vi "Chamber controller Dec 14 2016.vi"() -> ()   [LabVIEW 2014]
uses:
  <vilib>/Instr/_visa.llb/VISA Configure Serial Port (Instr).vi
  Environmental Chamber LabVIEW and Instruments/Drivers and Software/Keithley 2100 Series/Public/Configure/Configure 2 Wire Resistance.vi
  <vilib>/Utility/file.llb/Write To Spreadsheet File (string).vi
  <vilib>/Utility/file.llb/Read From Spreadsheet File (string).vi
  Environmental Chamber LabVIEW and Instruments/Drivers and Software/keithley_6430/Keithley 6430/Public/Data/Read (Single Point).vi
  Environmental Chamber LabVIEW and Instruments/Drivers and Software/LabVIEW 8.2 Drivers/keithley_24xx/Keithley 24XX/Public/Data/Read (Single Point).vi
  Environmental Chamber LabVIEW and Instruments/Drivers and Software/keithley_24xx/Keithley 24XX/Keithley 24XX.lvlib
  Environmental Chamber LabVIEW and Instruments/Drivers and Software/keithley_6430/Keithley 6430/Keithley 6430.lvlib
  Environmental Chamber LabVIEW and Instruments/Drivers and Software/Keithley 2100 Series/Keithley 2100 Series.lvlib
panel:
  in  "Pressure parameters cluster":T1={"valve % open"=100.0, "Desired pressure"=0.0, "Vapor sccm"=0.0, "Gas sccm"=0.0, "Valve mode"=enum."% Open", "Pressure Mode"=enum."Abs. pressure", "analyte partial pressure"=23.8, "Turbo pump\nauto on"=TRUE, "Valve position (%)"=0.0, "read pressure"=0.0, "read vapor flow"=0.0, "read gas flow"=0.0} caption="Pressure settings" {"read gas flow" format="%#_3g"; "read vapor flow" format="%#_3g"; "read pressure" format="%#_7f"; "Valve position (%)" format="%#_3g"; "analyte partial pressure" min=0.0 max=100.0 step=5.0; "Gas sccm" min=0 max=200 step=5; "Vapor sccm" min=0 max=200 step=5; "Desired pressure" min=0.0 max=760.0 step=5.0; "valve % open" min=0.0 max=100.0 step=5.0 format="%#_2f"}
  out "pressure chart":cluster{"pressure":dbl}(graph)
  out "arduino qcm stack plot":T2(graph)
  in  "K-2420 tab control":enum32{"K-2420 Measure", "K-2420 Apply bias"}(tab)
  out "K-2420 2":cluster{"Resistance":sgl}(graph)
  in  "Bias (V)":dbl min=-5.0 max=5.0 step=5e-06
  out "K-2420 4":cluster{"Applied Voltage (V)":dbl}(graph)
  out "saving data?":bool
  in  "Data logging settings":T3={"Save during sequence only"=TRUE, "Save now"=FALSE, "sec between points"=0.0, "Current data file path"=path "", "Save sample/gas names"={"QCM1"="", "QCM2"="", "QCM3"="", "QCM4"="", "QCM5"="", "QCM6"="", "SRS"="bareAu", "K-2420"="", "K-6430"="", "K-2100"="", "Gas"="O2", "Vapor"="H2O"}, "add notes to file"=FALSE} {"sec between points" min=0.0 max=30.0 format="%#_13g"}
  in  "Sequence cluster":T4={"Save sequence"=FALSE, "Clear sequence"=FALSE, "Import sequence file"=FALSE, "Run Sequence"=FALSE, "Stop program when sequence ends"=TRUE, "User-defined\nsequence"=[], "Sequence end time"="", "Sequence\npreview"=[], "Current\nstep"=0, "Display"=0, "Sequence length (hrs)"=0.0} caption="Pressure settings" {"Display" items=["pressure", "gas flow", "vapor flow", "bias"]}
  out "J-KEM temp chart":dbl(graph)
  out "State date/time":string caption="Start time"
  out "K-2100 (Ohm)":cluster{"Measurement":dbl}(graph) caption="K-2100"
  out "K-6430":cluster{"Measurement":dbl}(graph)
  in  "Gate time (s)":enum16{"0.1", "1.0 ", "10"}(ring)=enum."1.0 "
  out "Hz":dbl format="%#.7f"
  out "QCM plot":T5(graph)
  in  "Stop":bool
  in  "Clear all charts":bool
  out "O2 sensor output":dbl[](array[numeric]) caption="atm\nTorr"
  in  "rapidox O2 Sensor":bool
  in  "setnag O2 Pump":bool
  in  "Baud Rate 2":i32(ring)=2 items=["2400", "4800", "9600", "19200", "38400", "57600", "115200"]
  in  "Com Port":i32(ring) items=["Com 1", "Com 2", "Com 3", "Com 4", "Com 5", "Com 6", "COM 7", "COM 8", "COM 9", "COM 10", "COM 11", "COM 12", "com 13", "COM 14"]
  in  "Com Port 2":i32(ring) items=["Com 1", "Com 2", "Com 3", "Com 4", "Com 5", "Com 6", "COM 7", "COM 8", "COM 9", "COM 10", "COM 11", "COM 12", "com 13", "COM 14"]
  out "Waveform Chart":cluster{dbl}(graph)
  out "O2 Concentration (PPM)":dbl
  out "Waveform Chart 6":cluster{dbl}(graph)
  # "SRS"
  # "Currently Unused"
  # "100%"
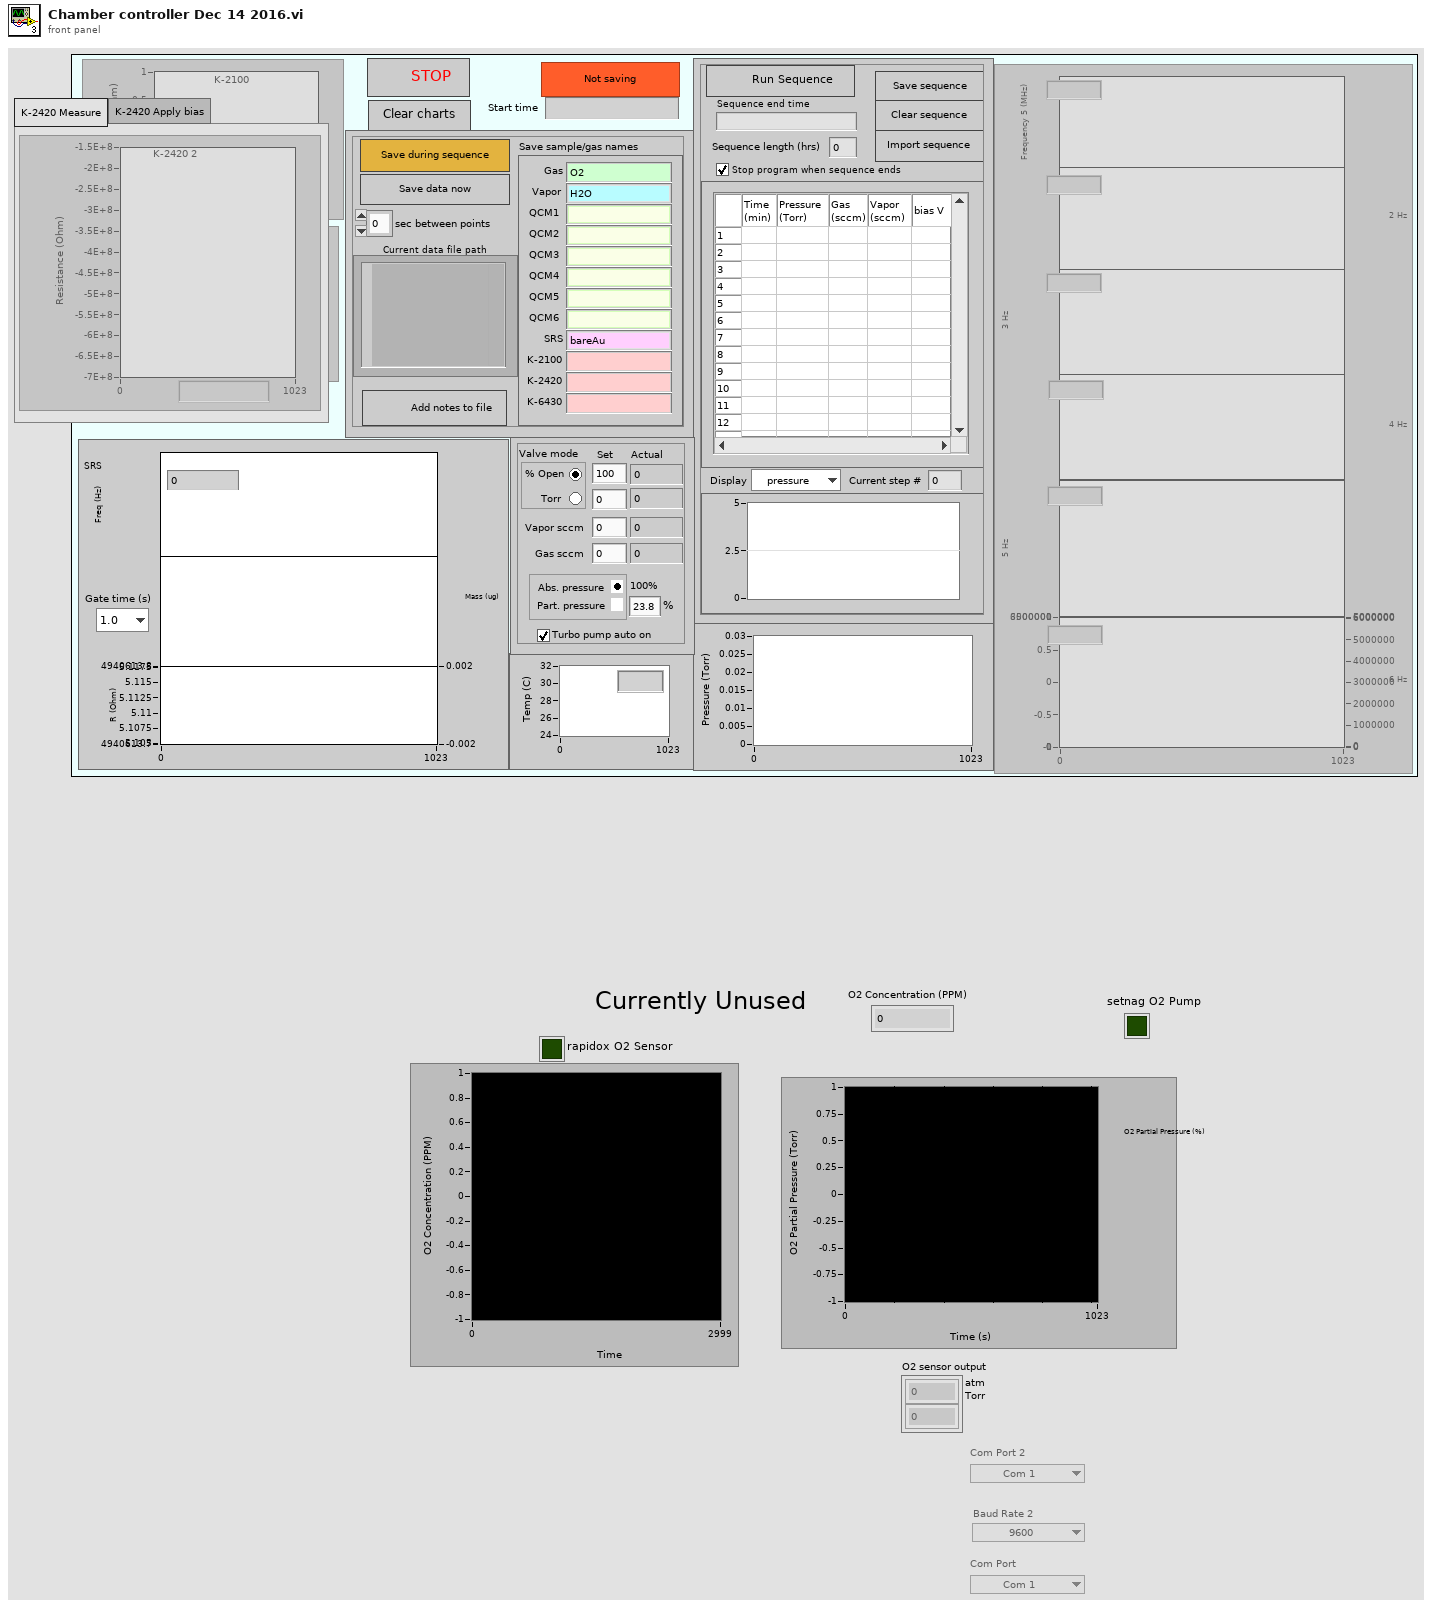
[diagram p1: front panel]
types:
  T1 = cluster{"valve % open":dbl, "Desired pressure":dbl, "Vapor sccm":sgl, "Gas sccm":sgl, "Valve mode":enum32{"% Open", "Torr "}, "Pressure Mode":enum32{"Abs. pressure", " Part. pressure"}, "analyte partial pressure":dbl, "Turbo pump\nauto on":bool, "Valve position (%)":dbl, "read pressure":dbl, "read vapor flow":dbl, "read gas flow":dbl}
  T2 = cluster{"mean":dbl, "mean":dbl, "mean":dbl, "mean":dbl, "mean":dbl, "mean":dbl}
  T3 = cluster{"Save during sequence only":bool, "Save now":bool, "sec between points":dbl, "Current data file path":path, "Save sample/gas names":cluster{"QCM1":string, "QCM2":string, "QCM3":string, "QCM4":string, "QCM5":string, "QCM6":string, "SRS":string, "K-2420":string, "K-6430":string, "K-2100":string, "Gas":string, "Vapor":string}, "add notes to file":bool}
  T4 = cluster{"Save sequence":bool, "Clear sequence":bool, "Import sequence file":bool, "Run Sequence":bool, "Stop program when sequence ends":bool, "User-defined\nsequence":string[][], "Sequence end time":string, "Sequence\npreview":cluster{dbl[], dbl[]}[], "Current\nstep":i32, "Display":u16, "Sequence length (hrs)":dbl}
  T5 = cluster{"Frequency out":dbl, "Numeric Control":dbl, "Resistance out":dbl}
  T6 = cluster{"Keithley 6430":bool, "J-KEM":bool, "Keithley 2420":bool, "Keithley 2100":bool, "SRS QCM":bool, "Pressure control":bool, "Arduino":bool}
  T7 = cluster{"Arduino 1":refnum<visa-resource-name>, "Arduino 2":refnum<visa-resource-name>, "Arduino 3":refnum<visa-resource-name>, "Arduino 4":refnum<visa-resource-name>, "Arduino 5":refnum<visa-resource-name>, "Arduino 6":refnum<visa-resource-name>}
  T8 = enum8{"Enabled", "Disabled", "Disabled and Grayed Out"}
  T9 = enum16{"open", "open or create", "create or replace", "create", "open (read only)"}
  T10 = enum16{"no parity", "odd parity", "even parity", "mark parity", "space parity"}
  T11 = cluster{"mean":dbl, "mean":dbl, "mean":dbl, "mean":dbl, "mean":dbl, "mean":dbl}[]
  T12 = cluster{"Frequency out":dbl, "Numeric Control":dbl, "Resistance out":dbl}[]
  T13 = cluster{"String":string, "String":string, "String":string}
  T14 = cluster{bool, "task out":refnum<k21>, "error out":errorcluster, "task out":refnum<k21>, "error out":errorcluster, "turbo pump":refnum<visa-resource-name>, "error out":errorcluster}
  T15 = cluster{bool, "task out":refnum<k21>, "error out":errorcluster, "task out":refnum<k21>, "error out":errorcluster, "VISA resource name out":refnum<visa-resource-name>, "error out":errorcluster}
  T16 = cluster{bool, "VISA resource name":refnum<visa-resource-name>, "error out":errorcluster}
  T17 = cluster{bool, "VISA resource name out":refnum<visa-resource-name>, "error out":errorcluster}
  T18 = cluster{"VISA resource name out":refnum<visa-resource-name>, "error out":errorcluster, "VISA resource name out":refnum<visa-resource-name>, "error out":errorcluster, "VISA resource name out":refnum<visa-resource-name>, "error out":errorcluster, "VISA resource name out":refnum<visa-resource-name>, "error out":errorcluster, "VISA resource name out":refnum<visa-resource-name>, "error out":errorcluster, "VISA resource name out 2":refnum<visa-resource-name>, "error out 2":errorcluster}
  T19 = cluster{"Boolean":bool, "VISA resource name out":refnum<visa-resource-name>, "error out":errorcluster}
  T20 = cluster{bool, "VISA out":refnum<visa-resource-name>, "error out":errorcluster}
  T21 = cluster{"Boolean":bool, "VISA out":refnum<visa-resource-name>, "error out":errorcluster}
  T22 = cluster{"Numeric Control":dbl, "Cluster":cluster{"Numeric Control":dbl}, "String":string, "error out":errorcluster}
  T23 = cluster{bool, "Com Port":i32, "Numeric Control out":dbl}
  T24 = cluster{"Arduino address":refnum<visa-resource-name>, "error in (no error)":errorcluster, "Arduino address 2":refnum<visa-resource-name>, "error in (no error) 2":errorcluster, "Arduino address 3":refnum<visa-resource-name>, "error in (no error) 3":errorcluster, "Arduino address 4":refnum<visa-resource-name>, "error in (no error) 4":errorcluster, "Arduino address 5":refnum<visa-resource-name>, "error in (no error) 5":errorcluster, "Arduino address 6":refnum<visa-resource-name>, "error in (no error) 6":errorcluster}
  T25 = cluster{"mean":string, "mean":string, "mean":string, "mean":string, "mean":string, "mean":string}
  T26 = cluster{"valve % open":dbl, "Desired pressure":dbl, "Vapor sccm":sgl, "Gas sccm":sgl, "Valve mode":enum32{"% Open", "Torr "}, "Pressure Mode":enum32{"Abs. pressure", " Part. pressure"}, "analyte partial pressure":dbl}
  T27 = cluster{"User-defined\nsequence":string[][], "Present (s)":dbl, "current  step # in":i32, "sequence end time in":timestamp}
  T28 = cluster{"current  step # in":i32, "sequence end time in":timestamp, "Boolean":bool}
  T29 = cluster{"press/RH/gas/vapor":cluster{"pressure":string, "RH":string, "gas flow":string, "vapor flow":string}, "Cluster":cluster{"Valve position (%)":dbl, "read pressure":dbl, "read vapor flow":dbl, "read gas flow":dbl}}
  T30 = cluster{"Boolean":bool, "task out":refnum<k21>, "error out":errorcluster, "task out":refnum<k21>, "error out":errorcluster, "VISA resource name out":refnum<visa-resource-name>, "error out":errorcluster}
  T31 = cluster{"pressure":string, "RH":string, "gas flow":string, "vapor flow":string}
  T32 = cluster{"Valve position (%)":dbl, "read pressure":dbl, "read vapor flow":dbl, "read gas flow":dbl}
  T33 = cluster{"f":dbl, "f":dbl, "f":dbl, "f":dbl, "f":dbl}[]
  T34 = cluster{"QCM1":string, "QCM2":string, "QCM3":string, "QCM4":string, "QCM5":string, "QCM6":string, "SRS":string, "K-2420":string, "K-6430":string, "K-2100":string, "Gas":string, "Vapor":string}
  T35 = cluster{"String data out":string, string, string, string}
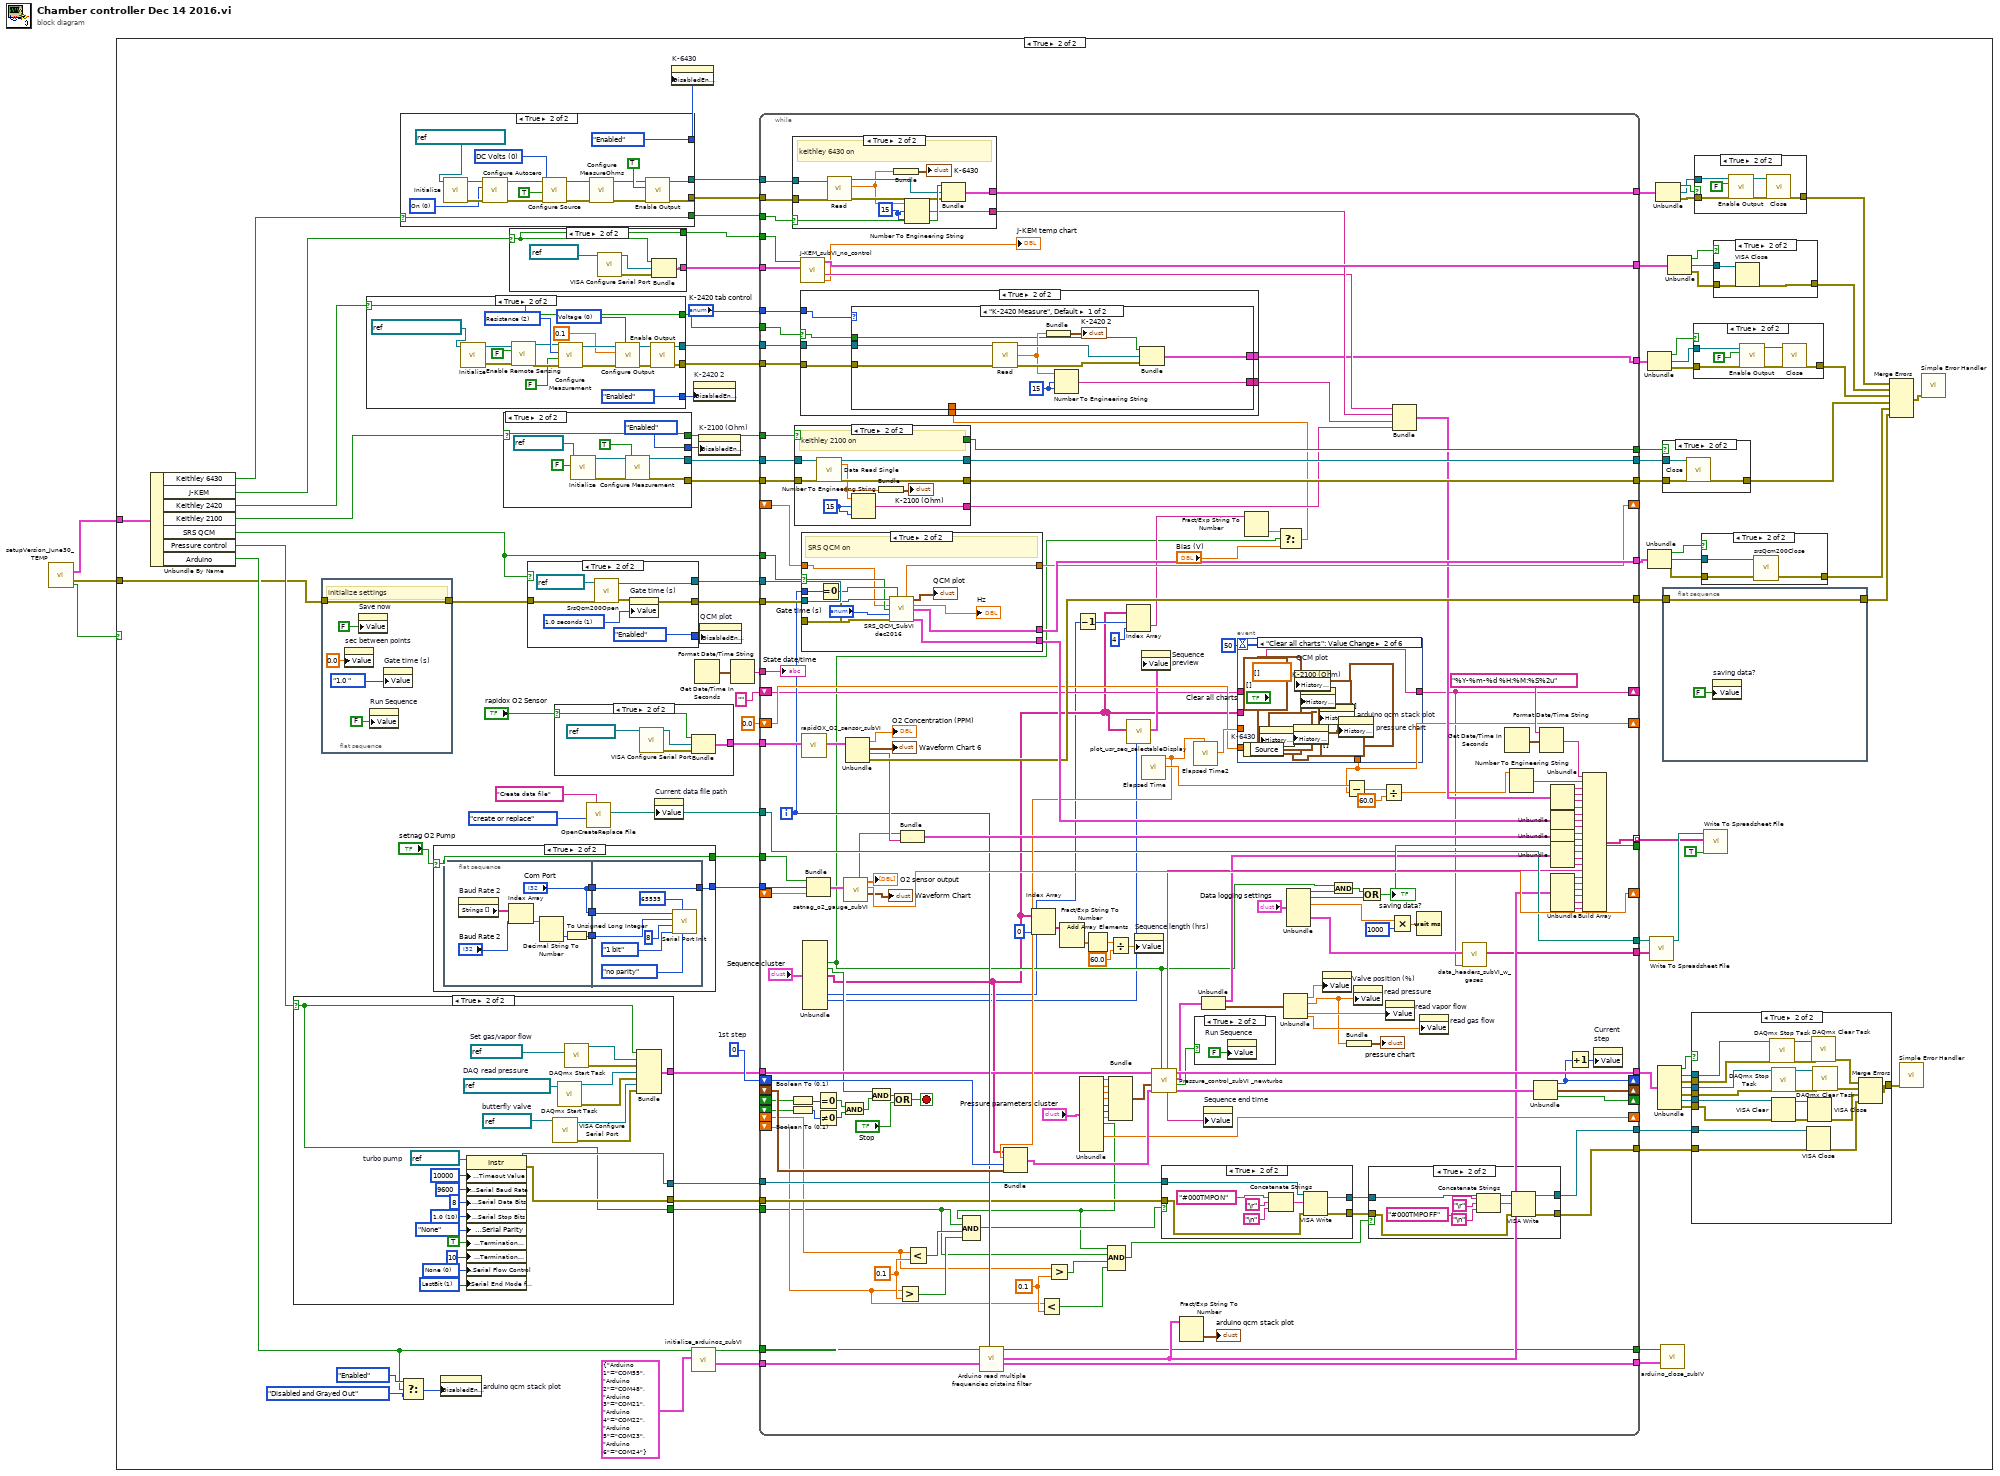
[diagram p0: block diagram]
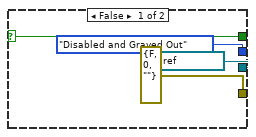
[diagram p4: hidden frame]
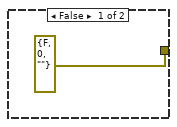
[diagram p5: hidden frame]
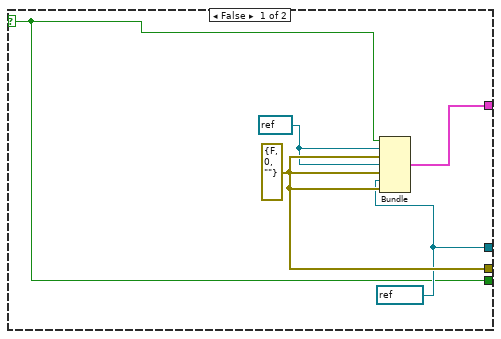
[diagram p6: hidden frame]
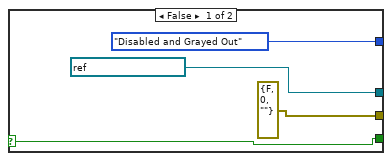
[diagram p8: hidden frame]
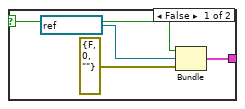
[diagram p9: hidden frame]
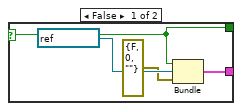
[diagram p11: hidden frame]
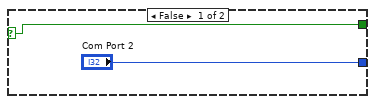
[diagram p12: hidden frame]
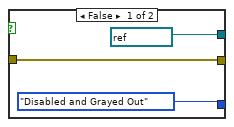
[diagram p14: hidden frame]
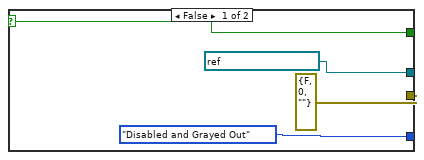
[diagram p16: hidden frame]
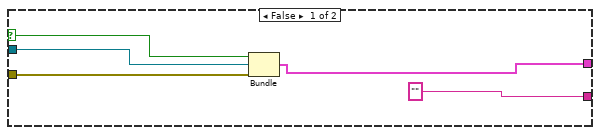
[diagram p17: hidden frame]
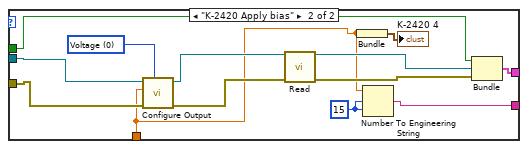
[diagram p18: hidden frame]
diagram:
  n1 = call "setupVersion_June30_TEMP.vi"() -> ("Instruments on/off"=w1:T6, "error IO"=w2:errorcluster, "OK"=w3:bool)  [unwired: 13 in]
  n2 = case shown="True" w3 {
    tunnel: w2 -> [_ w22]
    tunnel: w1 -> [_ w32]
    frame False {
    }
    frame True {
      w38 = 0  # 1st step
      n3 = Unbundle By Name(w32) -> ("Keithley 6430"=w31:bool, "J-KEM"=w30:bool, "Keithley 2420"=w29:bool, "Keithley 2100"=w28:bool, "SRS QCM"=w27:bool, "Pressure control"=w26:bool, "Arduino"=w25:bool)
      n4 = case shown="True" w26 {
        selector: w26 -> [w144 w149]
        tunnel: [w148 w150] -> w20
        tunnel: [w147 w152] -> w12
        tunnel: [w145 w151] -> w13
        tunnel: [w144 w149] -> w11
        frame False {
          w145 = refnum<visa-resource-name> refnum ("turbo pump")
          w146 = refnum<k21> refnum ("task out")
          w147 = errorcluster {"status"=FALSE, "code"=0, "source"=""} ("error out")
          n5 = Bundle(w144, "task out"=w146, "error out"=w147, "task out"=w146, "error out"=w147, "turbo pump"=w145, "error out"=w147) -> (w148:T14)  [unwired: 1 in]
        }
        frame True {
          w156 = u16 1 items=["None", "LastBit", "TermChar"] ("Serial Settings:Serial End Mode for Reads")
          w154 = u16 0 items=["None", "XON/XOFF", "RTS/CTS", "XON/XOFF & RTS/CTS", "DTR/DSR", "XON/XOFF & DTR/DSR"] ("flow control (0:none)")
          w157 = u16 10 items=["1.0"=10, "1.5"=15, "2.0"=20] ("stop bits (10: 1 bit)")
          w153 = refnum<visa-resource-name> "COM7"  # turbo pump
          w169 = refnum<visa-resource-name> "COM5"  # butterfly valve
          w170 = refnum<k21> "Setflow"  # Set gas/vapor flow
          w171 = refnum<k21> "AllDaqReadings"  # DAQ read pressure
          n6 = property class="Instr"(reference=w153, "General Settings:Timeout Value"=u32 10000 ("timeout (10sec)"), "Serial Settings:Serial Baud Rate"=u32 9600 ("baud rate (9600)"), "Serial Settings:Serial Data Bits"=u16 8 ("data bits (8)"), "Serial Settings:Serial Stop Bits"=w157, "Serial Settings:Serial Parity"=enum16{"None", "Odd", "Even", "Mark", "Space"}."None" ("parity (0:none)"), "Message Based Settings:Termination Character Enable"=TRUE ("Enable Termination\nChar (T)"), "Message Based Settings:Termination Character"=u8 10 ("termination char\n(0xA = '\\n' = LF)"), "Serial Settings:Serial Flow Control"=w154, "Serial Settings:Serial End Mode for Reads"=w156) -> (reference out=w151:refnum<visa-resource-name>, error out=w152:errorcluster)  [unwired: 1 in]
          n7 = call-poly "VISA Configure Serial Port"("VISA resource name"=w169) -> ("VISA resource name out"=w164:refnum<visa-resource-name>, "error out"=w163:errorcluster)  [unwired: 13 in]
          n8 = call <vilib>:"DAQmx Start Task.vi"("task/channels in"=w171) -> ("task out"=w166:refnum<k21>, "error out"=w165:errorcluster)  [unwired: 13 in]
          n9 = call <vilib>:"DAQmx Start Task.vi"("task/channels in"=w170) -> ("task out"=w168:refnum<k21>, "error out"=w167:errorcluster)  [unwired: 13 in]
          n10 = Bundle(w149, "task out"=w168, "error out"=w167, "task out"=w166, "error out"=w165, "VISA resource name out"=w164, "error out"=w163) -> (w150:T15)  [unwired: 1 in]
        }
      }
      n11 = flat-sequence {
        tunnel: [w100] -> w21
        tunnel: w22 -> [w100]
        frame #0 {
          # "initialize settings"
          n12 = property on="sec between points" class="DigNum (strict)"("Value"=0.0) -> ()  [unwired: 2 in, 2 out]
          n13 = property on="Save now" class="Bool (strict)"("Value"=FALSE) -> ()  [unwired: 2 in, 2 out]
          n14 = property on="Run Sequence" class="Bool (strict)"("Value"=FALSE) -> ()  [unwired: 2 in, 2 out]
          n15 = property on="Gate time (s)" class="Enum (strict)"("Value"=enum16{"0.1", "1.0 ", "10"}."1.0 " ("Gate time (sec)")) -> ()  [unwired: 2 in, 2 out]
        }
      }
      n16 = case shown="True" w29 {
        selector: w29 -> [w263 w267]
        tunnel: [refnum<visa-resource-name> "GPIB1::24::INSTR" ("VISA resource name") w276] -> w97
        tunnel: [errorcluster {"status"=FALSE, "code"=0, "source"=""} ("error out") w271] -> w96
        tunnel: [T8."Disabled and Grayed Out" ("Disabled") T8."Enabled" ("Disabled")] -> w4
        tunnel: [w263 w267] -> w54
        frame False {
        }
        frame True {
          w278 = u16 0 items=["Voltage", "Current"] ("Source Mode  (0: Voltage)")
          w283 = u16 2 items=["Volts", "Current", "Resistance"] ("Function (0: Volts)")
          n17 = call "Initialize.vi"("VISA resource name"=refnum<visa-resource-name> "GPIB1::24::INSTR") -> ("error out"=w272:errorcluster, "VISA resource name out"=w275:refnum<visa-resource-name>)  [unwired: 9 in]
          n18 = call "Enable Remote Sensing.vi"("error in (no error)"=w272, "Enable Remote Sensing (T: Enable)"=FALSE ("4-wire?"), "VISA resource name"=w275) -> ("error out"=w273:errorcluster, "VISA resource name out"=w274:refnum<visa-resource-name>)  [unwired: 7 in]
          n19 = call "Configure Measurement.vi"("error in (no error)"=w273, "Enable Auto Range (T:Enable)"=FALSE, "Function (0: Volts)"=w283, "VISA resource name"=w274) -> ("error out"=w282:errorcluster, "VISA resource name out"=w281:refnum<visa-resource-name>)  [unwired: 6 in]
          n20 = call "Configure Output.vi"("Source Mode  (0: Voltage)"=w278, "error in (no error)"=w282, "Output Level (0)"=0.1 ("Applied Voltage (V)"), "VISA resource name"=w281) -> ("error out"=w280:errorcluster, "VISA resource name out"=w279:refnum<visa-resource-name>)  [unwired: 6 in]
          n21 = call "Enable Output.vi"("error in (no error)"=w280, "VISA resource name"=w279) -> ("error out"=w271:errorcluster, "VISA resource name out"=w276:refnum<visa-resource-name>)  [unwired: 8 in]
        }
      }
      n22 = case shown="True" w31 {
        selector: w31 -> [w179 w183]
        tunnel: [refnum<visa-resource-name> "GPIB0::29::INSTR" ("VISA resource name") w194] -> w66
        tunnel: [errorcluster {"status"=FALSE, "code"=0, "source"=""} ("error out") w195] -> w65
        tunnel: [T8."Disabled and Grayed Out" ("Disabled") T8."Enabled" ("Disabled")] -> w60
        tunnel: [w179 w183] -> w53
        frame False {
        }
        frame True {
          w184 = u16 0 items=["DC Volts", "DC Current"] ("Source Function (0: DC Volts)")
          w191 = u16 0 items=["On", "Off", "Once"] ("Autozero  (0: On)")
          n23 = call "Initialize.vi"("VISA resource name"=refnum<visa-resource-name> "GPIB0::29::INSTR") -> ("error out"=w192:errorcluster, "VISA resource name out"=w193:refnum<visa-resource-name>)  [unwired: 4 in, 5 out]
          n24 = call "Configure Autozero.vi"("error in (no error)"=w192, "Autozero  (0: On)"=w191, "VISA resource name"=w193) -> ("error out"=w187:errorcluster, "VISA resource name out"=w189:refnum<visa-resource-name>)  [unwired: 7 in]
          n25 = call "Configure Source.vi"("error in (no error)"=w187, "Auto Range (T:Enable)"=TRUE, "Source Function (0: DC Volts)"=w184, "VISA resource name"=w189) -> ("error out"=w186:errorcluster, "VISA resource name out"=w188:refnum<visa-resource-name>)  [unwired: 6 in]
          n26 = call "Configure MeasureOhms.vi"("error in (no error)"=w186, "VISA resource name"=w188) -> ("error out"=w199:errorcluster, "VISA resource name out"=w197:refnum<visa-resource-name>)  [unwired: 4 in, 4 out]
          n27 = call "Enable Output.vi"("error in (no error)"=w199, "Enable Output (F:Off)"=TRUE ("Output (F:Off)"), "VISA resource name"=w197) -> ("error out"=w195:errorcluster, "VISA resource name out"=w194:refnum<visa-resource-name>)  [unwired: 7 out]
        }
      }
      n28 = Select(t=T8."Enabled" ("Disabled"), s=w25, f=T8."Disabled and Grayed Out" ("Disabled")) -> (s? t:f=w6:T8)
      n29 = case shown="True" "setnag O2 Pump" {
        selector: "setnag O2 Pump" -> [w222 w224]
        tunnel: ["Com Port 2" w225] -> w93
        tunnel: [w222 w224] -> w43
        frame False {
        }
        frame True {
          n30 = flat-sequence {
            tunnel: ["Com Port"] -> w228
            tunnel: [w230] -> w227
            tunnel: ["Com Port"] -> w226
            tunnel: w228 -> [w236]
            tunnel: w227 -> [w235]
            tunnel: w226 -> [w237]
            tunnel: [w237] -> w225
            frame #0 {
              n31 = property on="Baud Rate 2" class="Ring (strict)"() -> ("Strings []"=w232:string[])  [unwired: 2 in, 2 out]
              n32 = Index Array(array=w232, index="Baud Rate 2") -> (element=w233:string)
              n33 = Decimal String To Number(string=w233) -> (number=w231:i32)  [unwired: 2 in, 1 out]
              n34 = To Unsigned Long Integer(number=w231) -> (unsigned 32bit integer=w230:u32)
            }
            frame #1 {
              n35 = call <vilib>:"Serial Port Init.vi"("parity"=T10."no parity", "buffer size"=u16 65535, "stop bits"=enum16{"1 bit", "1.5 bits", "2 bits"}."1 bit", "data bits"=u16 8, "baud rate"=w235, "port number"=w236) -> ()  [unwired: 1 in, 1 out]
            }
          }
        }
      }
      n36 = property on="arduino qcm stack plot" class="WFChart (strict)"("DisabledEnum"=w6) -> ()  [unwired: 2 in, 2 out]
      n37 = case shown="True" w28 {
        selector: w28 -> [w112 w117]
        tunnel: [refnum<visa-resource-name> "K-2100" ("VISA resource name out") w120] -> w52
        tunnel: [errorcluster {"status"=FALSE, "code"=0, "source"=""} ("error out") w119] -> w51
        tunnel: [w112 w117] -> w50
        tunnel: [T8."Disabled and Grayed Out" ("Disabled") T8."Enabled" ("Disabled")] -> w45
        frame False {
        }
        frame True {
          n38 = call "Initialize.vi"("VISA resource name"=refnum<visa-resource-name> "K-2100", "Reset? (T: Reset)"=FALSE) -> ("VISA resource name out"=w121:refnum<visa-resource-name>, "error out"=w118:errorcluster)  [unwired: 16 in]
          n39 = call-poly "Configure Measurement.vi"("VISA resource name"=w121, "error in (no error)"=w118, "Auto Range? (T: Auto)"=TRUE) -> ("VISA resource name out"=w120:refnum<visa-resource-name>, "error out"=w119:errorcluster)  [unwired: 15 in]
        }
      }
      n40 = case shown="True" w30 {
        selector: w30 -> [w213 w218]
        tunnel: [w214 w219] -> w82
        tunnel: [w213 w218] -> w76
        frame False {
          n41 = Bundle(w213, "VISA resource name"=refnum<visa-resource-name> "COM3", "error out"=errorcluster {"status"=FALSE, "code"=0, "source"=""}) -> (w214:T16)  [unwired: 1 in]
        }
        frame True {
          n42 = call-poly "VISA Configure Serial Port"("VISA resource name"=refnum<visa-resource-name> "COM3") -> ("VISA resource name out"=w220:refnum<visa-resource-name>, "error out"=w217:errorcluster)  [unwired: 13 in]
          n43 = Bundle(w218, "VISA resource name out"=w220, "error out"=w217) -> (w219:T17)  [unwired: 1 in]
        }
      }
      n44 = case shown="True" w27 {
        tunnel: [refnum<visa-resource-name> "COM6" ("VISA in") w252] -> w95
        tunnel: [w247 w249] -> w94
        tunnel: w21 -> [w247 w254]
        tunnel: [T8."Disabled and Grayed Out" ("Disabled") T8."Enabled" ("Disabled")] -> w61
        frame False {
        }
        frame True {
          w251 = u16 1 items=["0.1 seconds", "1.0 seconds", "10.0 seconds"] ("Gate time")
          n45 = call "SrsQcm200Open.vi"("error in"=w254, "VISA in"=refnum<visa-resource-name> "COM6") -> ("error out"=w250:errorcluster, "VISA out"=w252:refnum<visa-resource-name>)  [unwired: 3 in]
          n46 = property on="Gate time (s)" class="Enum (strict)"(error in=w250, "Value"=w251) -> (error out=w249:errorcluster)  [unwired: 1 in, 1 out]
        }
      }
      n47 = case shown="True" "rapidox O2 Sensor" {
        selector: "rapidox O2 Sensor" -> [w200 w205]
        tunnel: [w201 w206] -> w72
        frame False {
          n48 = Bundle(w200, "VISA resource name"=refnum<visa-resource-name> "COM7", "error out"=errorcluster {"status"=FALSE, "code"=0, "source"=""}) -> (w201:T16)  [unwired: 1 in]
        }
        frame True {
          n49 = call-poly "VISA Configure Serial Port"("VISA resource name"=refnum<visa-resource-name> "COM7") -> ("VISA resource name out"=w207:refnum<visa-resource-name>, "error out"=w204:errorcluster)  [unwired: 13 in]
          n50 = Bundle(w205, "VISA resource name out"=w207, "error out"=w204) -> (w206:T17)  [unwired: 1 in]
        }
      }
      n51 = call "OpenCreateReplace File.vi"("prompt"="Create data file", "function (open:0)"=T9."create or replace") -> ("new file path"=w8:path)  [unwired: 6 in, 3 out]
      n52 = property on="Current data file path" class="Path"("Value"=w8) -> ()  [unwired: 2 in, 2 out]
      n53 = property on="K-6430" class="WFChart (strict)"("DisabledEnum"=w60) -> ()  [unwired: 2 in, 2 out]
      n54 = call "initialize_arduinos_subVI.vi"("arduino 1-6 addresses"=T7 {"Arduino 1"="COM55", "Arduino 2"="COM48", "Arduino 3"="COM21", "Arduino 4"="COM22", "Arduino 5"="COM23", "Arduino 6"="COM24"} ("Arduino COMs"), "arduinos on?"=w25) -> ("arduino addresses/errors"=w39:T18, "arduinos on/off"=w58:bool)  [unwired: 8 in]
      n55 = property on="K-2420 2" class="WFChart (strict)"("DisabledEnum"=w4) -> ()  [unwired: 2 in, 2 out]
      n56 = Get Date/Time In Seconds() -> (seconds since 1Jan1904=w99:timestamp)
      n57 = property on="K-2100 (Ohm)" class="WFChart (strict)"("DisabledEnum"=w45) -> ()  [unwired: 2 in, 2 out]
      n58 = property on="QCM plot" class="WFChart (strict)"("DisabledEnum"=w61) -> ()  [unwired: 2 in, 2 out]
      n59 = Format Date/Time String(seconds (now)=w99) -> (date/time string=w42:string)  [unwired: 2 in]
      n60 = while {
        shift-right: [w461] -> _
        shift-left: _ -> [w398]
        tunnel: [w449] -> w59 mode=indexing if=w419
        tunnel: w54 -> [w307]
        tunnel: w97 -> [w309]
        tunnel: w96 -> [w308]
        tunnel: w95 -> [w460]
        tunnel: w94 -> [w459]
        tunnel: w27 -> [w458]
        tunnel: w43 -> [w400]
        tunnel: w93 -> [w401]
        tunnel: [w302] -> w90
        tunnel: [w457] -> w86
        tunnel: w82 -> [w456]
        tunnel: [w455] -> w81
        tunnel: w76 -> [w454]
        tunnel: w72 -> [w408]
        tunnel: [w404] -> w24
        tunnel: [w349] -> w71
        tunnel: w8 -> [w349]
        shift-right: [w447] -> _
        shift-left: _ -> [w448]
        tunnel: w66 -> [w453]
        tunnel: w65 -> [w452]
        tunnel: [w451] -> w64
        tunnel: [w419] -> _
        tunnel: w58 -> [w338]
        tunnel: w39 -> [w341]
        tunnel: [w337] -> w56
        tunnel: [w339] -> w57
        tunnel: [w310] -> w55
        tunnel: w53 -> [w431]
        tunnel: w52 -> [w418]
        tunnel: w51 -> [w417]
        tunnel: w50 -> [w416]
        tunnel: [w415] -> w49
        tunnel: [w414] -> w48
        tunnel: [w413] -> w47
        shift-right: [w392] -> _
        shift-left: 0.0 ("Elapsed Time (s)") -> [w393]
        tunnel: w42 -> [w383]
        tunnel: w20 -> [w334]
        shift-right: [w346] -> _
        shift-left: w38 -> [w360]
        shift-right: [w365] -> _
        shift-left: _ -> [w363]
        shift-right: [w364] -> _
        shift-left: _ -> [w362]
        shift-left: _ -> [w361]
        tunnel: [w358] -> w37
        tunnel: w13 -> [w329]
        tunnel: w12 -> [w328]
        tunnel: w11 -> [w318]
        tunnel: [w323] -> w10
        tunnel: [w324] -> w9
        shift-right: [w333] -> _
        shift-left: _ -> [w320]
        shift-left: _ -> [w319]
        shift-right: [w299] -> _
        shift-left: "" ("notes to add") -> [w298]
        tunnel: "K-2420 tab control" -> [w285]
        i -> [w336]
        stop <- w421 stop-if-true
        w322 = 0.1 ("y")
        w332 = 0.1 ("y")
        n61 = Boolean To (0,1)(Boolean=w362) -> (0, 1=w429:i16)
        n62 = Boolean To (0,1)(Boolean=w361) -> (0, 1=w428:i16)
        n63 = case "Keithley 6430" shown="True" w431 {
          selector: w431 -> [w550 w561]
          tunnel: w453 -> [w549 w558]
          tunnel: w452 -> [w548 w557]
          tunnel: ["" w560] -> w403
          tunnel: [w547 w559] -> w451
          frame False {
            # "keithley 6430 off"
            n64 = Bundle(w550, "VISA resource name out"=w549, "error out"=w548) -> (w547:T17)  [unwired: 1 in]
          }
          frame True {
            w552 = i16 15 ("width (-)")
            # "keithley 6430 on"
            n65 = call-poly "Read.vi"("error in (no error)"=w557, "VISA resource name"=w558) -> ("error out"=w556:errorcluster, "Measurement"=w554:dbl, "VISA resource name out"=w555:refnum<visa-resource-name>)  [unwired: 1 in, 6 out]
            n66 = Bundle("Measurement"=w554) -> (→"K-6430":cluster{"Measurement":dbl})  [unwired: 1 in]
            n67 = Number To Engineering String(2:w552, 3:w552, 4:w554) -> (0:w560:string)  [unwired: 1 in]
            n68 = Bundle(w561, "VISA resource name out"=w555, "error out"=w556) -> (w559:T17)  [unwired: 1 in]
          }
        }
        n69 = case shown="True" w416 {
          selector: w416 -> [w519 w524]
          tunnel: [w520 w531] -> w414
          tunnel: [w521 w530] -> w413
          tunnel: w418 -> [w520 w529]
          tunnel: w417 -> [w521 w528]
          tunnel: ["" w526] -> w402
          tunnel: [w519 w524] -> w415
          frame False {
            # "keithley 2100 off"
          }
          frame True {
            w523 = i16 15 ("width (-)")
            # "keithley 2100 on"
            n70 = call "Data Read Single.vi"("VISA resource name"=w529, "error in (no error)"=w528) -> ("VISA resource name out"=w531:refnum<visa-resource-name>, "Measurement"=w527:dbl, "error out"=w530:errorcluster)  [unwired: 15 in]
            n71 = Number To Engineering String ("elapsed time (min)")(2:w523, 3:w523, 4:w527) -> (0:w526:string)  [unwired: 1 in]
            n72 = Bundle("Measurement"=w527) -> (→"K-2100 (Ohm)":cluster{"Measurement":dbl})  [unwired: 1 in]
          }
        }
        n73 = call "J-KEM_subVI_no_control.vi"("Address in"=w456, "J-KEM on?"=w454) -> ("Temp (C)"=→"J-KEM temp chart":dbl, "String data out"=w391:string, "Address out"=w455:T19)  [unwired: 6 in, 1 out]
        n74 = case "SRS QCM" shown="True" w458 {
          selector: w458 -> [w564 w574]
          tunnel: w460 -> [w567 w576]
          tunnel: w459 -> [w566 w578]
          tunnel: [w565 w571] -> w457
          tunnel: w448 -> [w562 w572]
          tunnel: [w562 w573] -> w447
          tunnel: [T13 {"String"="", "String"="", "String"=""} ("M,F,MR output cluster") w570] -> w440
          tunnel: w336 -> [_ w579]
          frame False {
            # "SRS QCM off"
            n75 = Bundle(w564, "VISA out"=w567, "error out"=w566) -> (w565:T20)  [unwired: 1 in]
          }
          frame True {
            # "SRS QCM on"
            n76 = Equal To 0?(x=w579) -> (x = 0?=w575:bool)
            n77 = call "SRS_QCM_SubVI  dec2016.vi"("VISA Refnum in"=w576, "first iteration?"=w575, "Frequency  in"=w572, "SRS on?"=w574, "Gate time"="Gate time (s)", "error in (no error)"=w578) -> ("Frequency out 2"=w573:dbl, "freq, mass, MR"=→"QCM plot":T5, "Frequency out"=→"Hz":dbl, "address out"=w571:T21, "M,F,MR output cluster"=w570:T13)  [unwired: 2 in, 3 out]
          }
        }
        n78 = call "rapidOX_O2_sensor_subVI.vi"("rapid ox info in"=w408) -> ("rapidox info out"=w407:T22)  [unwired: 10 in]
        n79 = Unbundle("Sequence cluster") -> ("Run Sequence"=w291:bool, "Stop program when sequence ends"=w290:bool, "User-defined\nsequence"=w289:string[][], "Current\nstep"=w288:i32, "Display"=w287:u16)  [unwired: 6 out]
        n80 = Bundle(w400, "Com Port"=w401, "Numeric Control out"=w398) -> (w399:T23)  [unwired: 1 in]
        n81 = Equal To 0?(x=w429) -> (x = 0?=w426:bool)
        n82 = Not Equal To 0?(x=w428) -> (x != 0?=w427:bool)
        n83 = And(x=w426, y=w427) -> (x .and. y?=w420:bool)
        n84 = call "setnag_o2_gauge_subVI.vi"("setnag info in"=w399) -> ("Cluster"=→"Waveform Chart":cluster{"Numeric Control":dbl}, "Numeric Control out"=w461:dbl, "Array"=→"O2 sensor output":dbl[], "String"=w347:string)  [unwired: 7 in]
        n85 = Unbundle(w407) -> ("Numeric Control"=→"O2 Concentration (PPM)":dbl, "Cluster"=→"Waveform Chart 6":cluster{"Numeric Control":dbl}, "String"=w382:string, "error out"=w404:errorcluster)
        n86 = And(x=w290, y=w420) -> (x .and. y?=w396:bool)
        n87 = Or(x=w396, y="Stop") -> (x .or. y?=w421:bool)
        n88 = Greater?(x=w319, y=w332) -> (0:w331:bool)
        n89 = Bundle("String"=w347, "String"=w382) -> (w381:cluster{"String":string, "String":string})  [unwired: 1 in]
        n90 = Less?(x=w320, y=w332) -> (x < y?=w330:bool)
        n91 = call "Arduino read multiple frequencies cristains filter.vi"("main loop iteration number"=w336, "arduino addresses in"=w341, "arduinos on?"=w338) -> ("arduino addresses out"=w339:T24, "arduino frequencies out"=w340:T25, "arduinos on"=w337:bool)  [unwired: 6 in]
        n92 = Index Array(array=w289, index (col)=0 ("disabled index (col)")) -> (element=w296:string[])  [unwired: 1 in]
        n93 = Less?(x=w319, y=w322) -> (x < y?=w316:bool)
        n94 = Greater?(x=w320, y=w322) -> (0:w317:bool)
        n95 = Fract/Exp String To Number(string=w296) -> (number=w295:dbl[])  [unwired: 3 in, 1 out]
        n96 = Decrement(x=w288) -> (x-1=w313:i32)
        n97 = Unbundle("Pressure parameters cluster") -> ("valve % open"=w372:dbl, "Desired pressure"=w373:dbl, "Vapor sccm"=w374:sgl, "Gas sccm"=w375:sgl, "Valve mode"=w376:enum32{"% Open", "Torr "}, "Pressure Mode"=w377:enum32{"Abs. pressure", " Part. pressure"}, "analyte partial pressure"=w378:dbl, "Turbo pump\nauto on"=w321:bool, "read pressure"=w333:dbl)  [unwired: 3 out]
        n98 = Compound Arithmetic op=AND(w321, w318, w330, w331) -> (w327:bool)
        n99 = Add Array Elements(numeric array=w295) -> (sum=w294:dbl)
        n100 = Compound Arithmetic op=AND(w321, w318, w317, w316) -> (w315:bool)
        n101 = Divide(x=w294, y=60.0) -> (x/y=w292:dbl)
        n102 = Bundle("valve % open"=w372, "Desired pressure"=w373, "Vapor sccm"=w374, "Gas sccm"=w375, "Valve mode"=w376, "Pressure Mode"=w377, "analyte partial pressure"=w378) -> (w371:T26)  [unwired: 1 in]
        n103 = Index Array(array=w289, index (row)=w313, index (col)=4 ("disabled index (col)")) -> (element=w304:string)
        n104 = call "plot_usr_seq_selectableDisplay.vi"("Display"=w287, "User-defined sequence"=w289) -> ("Sequence Preview"=w312:cluster{dbl[], dbl[]}[])  [unwired: 9 in]
        n105 = property on="Sequence length (hrs)" class="DigNum (strict)"("Value"=w292) -> ()  [unwired: 2 in, 2 out]
        n106 = property on="Sequence\npreview" class="XYGraph (strict)"("Value"=w312) -> ()  [unwired: 2 in, 2 out]
        n107 = call "Elapsed Time"() -> ("Present (s)"=w367:dbl, "Elapsed Time (s)"=w410:dbl)  [unwired: 12 in, 6 out]
        n108 = Bundle("User-defined\nsequence"=w289, "Present (s)"=w367, "current  step # in"=w360, "sequence end time in"=w363) -> (w368:T27)  [unwired: 1 in]
        n109 = call "Pressure_control_subVI _newturbo.vi"("Run Sequence"=w291, "user sequence, present (s) in, current step in, seq time in"=w368, "pressure parameters in"=w371, "pressure control on?/daq IDs/errors"=w334) -> ("current step # out, shift register time out, seq button on?"=w366:T28, "sequence over? USE THIS TO REINITIALIZE RUN SEQUENCE BUTTON SO PROGRAM ENDS"=w357:bool, "save press/RH/gasflow/vaporflow - read valve position/pressure/vaporflow/gasflow"=w356:T29, "pressure control on?/daq IDs/errors out"=w358:T30, "sequence end date/time string"=w359:string, "pressure_setpoint"=w343:string)  [unwired: 2 in]
        n110 = case shown="True" w327 {
          tunnel: w329 -> [w509 w512]
          tunnel: w328 -> [w508 w513]
          tunnel: [w509 w511] -> w326
          tunnel: [w508 w510] -> w325
          frame False {
          }
          frame True {
            n111 = Concatenate Strings("#000TMPON" ("write buffer 2"), "\r", "\n") -> (w514:string)
            n112 = VISA Write(VISA resource name=w512, write buffer=w514, error in (no error)=w513) -> (VISA resource name out=w511:refnum<visa-resource-name>, error out=w510:errorcluster)  [unwired: 1 out]
          }
        }
        n113 = Fract/Exp String To Number(string=w340) -> (number=→"arduino qcm stack plot":T2)  [unwired: 3 in, 1 out]
        n114 = call "Elapsed Time2"("Set Start Time (s)"=w367) -> ("Elapsed Time (s)"=w394:dbl)  [unwired: 11 in, 7 out]
        n115 = case shown="True" w357 {
          frame False {
          }
          frame True {
            n116 = property on="Run Sequence" class="Bool (strict)"("Value"=FALSE ("Run Sequence")) -> ()  [unwired: 2 in, 2 out]
          }
        }
        n117 = Unbundle(w356) -> ("press/RH/gas/vapor"=w355:T31, "Cluster"=w354:T32)
        n118 = property on="Sequence end time" class="Str"("Value"=w359) -> ()  [unwired: 2 in, 2 out]
        n119 = event shown="[1] \"Clear all charts\": Value Change" {
          selector: _ -> [_ _ _ _ _ _]
          dyn-events: _ -> [_ _ _ _ _ _]
          timeout: 50 -> [_ _ _ _ _ _]
          tunnel: w289 -> [_ _ _ _ w544 _]
          tunnel: w394 -> [_ _ _ _ _ _]
          tunnel: w393 -> [w533 _ _ _ _ _]
          tunnel: [w533 _ _ _ _ _] -> w392
          tunnel: [w532 w534 w540 w541 w543 w545] -> w299
          tunnel: w298 -> [w532 w534 w539 w541 w543 w545]
          event Timeout {
            n120 = event-data() -> ()  [unwired: 1 in, 1 out]
          }
          event "Clear all charts": Value Change {
            (unwired) T33 [] ("History Data")
            w537 = cluster{dbl}[] [] ("History Data")
            w538 = cluster{"Resistance":sgl}[] [] ("History Data")
            (unwired) dbl[] [] ("History Data")
            (unwired) cluster{dbl, "Resistance out":dbl}[] [] ("History Data")
            n121 = event-data() -> ()  [unwired: 1 in, 1 out]
            n122 = property on="K-6430" class="WFChart (strict)"("History Data"=w538) -> ()  [unwired: 2 in, 2 out]
            n123 = property on="Waveform Chart" class="WFChart (strict)"("History Data"=w537) -> ()  [unwired: 2 in, 2 out]
            n124 = property on="QCM plot" class="WFChart (strict)"("History Data"=T12 []) -> ()  [unwired: 2 in, 2 out]
            n125 = property on="K-2100 (Ohm)" class="WFChart (strict)"("History Data"=w538) -> ()  [unwired: 2 in, 2 out]
            n126 = property on="arduino qcm stack plot" class="WFChart (strict)"("History Data"=T11 []) -> ()  [unwired: 2 in, 2 out]
            n127 = property on="pressure chart" class="WFChart (strict)"("History Data"=w537) -> ()  [unwired: 2 in, 2 out]
          }
          event "Data logging settings.add notes to file": Value Change {
            n128 = event-data() -> ()  [unwired: 1 in, 1 out]
            n129 = call "notes_subVI.vi"("previous notes"=w539) -> ("notes to add"=w540:string)  [unwired: 14 in]
          }
          event "Sequence cluster.Clear sequence": Value Change {
            n130 = event-data() -> ()  [unwired: 1 in, 1 out]
            n131 = property on="User-defined\nsequence" class="Tbl (strict)"("Value"=string[][] []) -> ()  [unwired: 2 in, 2 out]
          }
          event "Sequence cluster.Save sequence": Value Change {
            n132 = event-data() -> ()  [unwired: 1 in, 1 out]
            n133 = call-poly <vilib>:"Write To Spreadsheet File.vi"("2D data"=w544) -> ()  [unwired: 7 in, 1 out]
          }
          event "Sequence cluster.Import sequence file": Value Change {
            n134 = event-data() -> ()  [unwired: 1 in, 1 out]
            n135 = call-poly <vilib>:"Read From Spreadsheet File.vi"() -> ("all rows"=w546:string[][])  [unwired: 7 in, 4 out]
            n136 = property on="User-defined\nsequence" class="Tbl (strict)"("Value"=w546) -> ()  [unwired: 2 in, 2 out]
          }
        }
        n137 = Fract/Exp String To Number(string=w304) -> (number=w303:dbl)  [unwired: 3 in, 1 out]
        n138 = Select(t=w303, s=w291, f="Bias (V)") -> (s? t:f=w306:dbl)
        n139 = case shown="True" w307 {
          selector: w307 -> [w467 w474]
          tunnel: ["" w473] -> w301
          tunnel: [w464 w472] -> w302
          tunnel: w309 -> [w466 w471]
          tunnel: w308 -> [w465 w470]
          tunnel: w306 -> [_ w469]
          tunnel: w285 -> [_ w468]
          frame False {
            n140 = Bundle(w467, "VISA resource name out"=w466, "error out"=w465) -> (w464:T17)  [unwired: 1 in]
          }
          frame True {
            n141 = case shown="\"K-2420 Measure\", Default" w468 {
              tunnel: w471 -> [w479 w491]
              tunnel: w470 -> [w478 w490]
              tunnel: [w477 w488] -> w472
              tunnel: w474 -> [w476 w489]
              tunnel: [w475 w487] -> w473
              tunnel: w469 -> [_ w486]
              frame "K-2420 Measure", Default {
                w480 = i16 15 ("width (-)")
                n142 = call-poly "Read.vi"("VISA resource name"=w479, "error in (no error)"=w478) -> ("VISA resource name out"=w483:refnum<visa-resource-name>, "Resistance"=w481:sgl, "error out"=w482:errorcluster)  [unwired: 7 in, 4 out]
                n143 = Bundle("Resistance"=w481) -> (→"K-2420 2":cluster{"Resistance":sgl})  [unwired: 1 in]
                n144 = Number To Engineering String(2:w480, 3:w480, 4:w481) -> (0:w475:string)  [unwired: 1 in]
                n145 = Bundle(w476, "VISA resource name out"=w483, "error out"=w482) -> (w477:T17)  [unwired: 1 in]
              }
              frame "K-2420 Apply bias" {
                w494 = u16 0 items=["Voltage", "Current"] ("Source Mode  (0: Voltage)")
                w495 = i16 15 ("width (-)")
                n146 = call "Configure Output.vi"("Source Mode  (0: Voltage)"=w494, "error in (no error)"=w490, "Output Level (0)"=w486, "VISA resource name"=w491) -> ("error out"=w492:errorcluster, "VISA resource name out"=w493:refnum<visa-resource-name>)  [unwired: 6 in]
                n147 = call-poly "Read.vi"("VISA resource name"=w493, "error in (no error)"=w492) -> ("VISA resource name out"=w497:refnum<visa-resource-name>, "error out"=w496:errorcluster)  [unwired: 7 in, 5 out]
                n148 = Bundle("Bias (V)"=w486) -> (→"K-2420 4":cluster{"Bias (V)":dbl})  [unwired: 1 in]
                n149 = Number To Engineering String(2:w495, 3:w495, 4:w486) -> (0:w487:string)  [unwired: 1 in]
                n150 = Bundle(w489, "VISA resource name out"=w497, "error out"=w496) -> (w488:T17)  [unwired: 1 in]
              }
            }
          }
        }
        n151 = Unbundle(w354) -> ("Valve position (%)"=w353:dbl, "read pressure"=w348:dbl, "read vapor flow"=w352:dbl, "read gas flow"=w351:dbl)
        n152 = Unbundle("Data logging settings") -> ("Save during sequence only"=w423:bool, "Save now"=w425:bool, "sec between points"=w412:dbl, "Save sample/gas names"=w311:T34)  [unwired: 2 out]
        n153 = property on="Valve position (%)" class="DigNum (strict)"("Value"=w353) -> ()  [unwired: 2 in, 2 out]
        n154 = And(x=w291, y=w423) -> (x .and. y?=w422:bool)
        n155 = Subtract(x=w410, y=w392) -> (x-y=w409:dbl)
        n156 = Bundle("read pressure"=w348) -> (→"pressure chart":cluster{"read pressure":dbl})  [unwired: 1 in]
        n157 = property on="read pressure" class="DigNum (strict)"("Value"=w348) -> ()  [unwired: 2 in, 2 out]
        n158 = Or(x=w422, y=w425) -> (x .or. y?=w419:bool)
        "saving data?" <- w419
        n159 = case shown="True" w315 {
          tunnel: w326 -> [w499 w502]
          tunnel: w325 -> [w498 w503]
          tunnel: [w499 w501] -> w323
          tunnel: [w498 w500] -> w324
          frame False {
          }
          frame True {
            n160 = Concatenate Strings("#000TMPOFF" ("write buffer 2"), "\r", "\n") -> (w504:string)
            n161 = VISA Write(VISA resource name=w502, write buffer=w504, error in (no error)=w503) -> (VISA resource name out=w501:refnum<visa-resource-name>, error out=w500:errorcluster)  [unwired: 1 out]
          }
        }
        n162 = Divide(x=w409, y=60.0) -> (x/y=w384:dbl)
        n163 = property on="read vapor flow" class="DigNum (strict)"("Value"=w352) -> ()  [unwired: 2 in, 2 out]
        n164 = Multiply(x=w412, y=u32 1000 ("x")) -> (x*y=w444:dbl)
        n165 = Bundle("String data out"=w391, w403, w301, w402) -> (w397:T35)  [unwired: 1 in]
        n166 = Wait (ms)(milliseconds to wait=w444) -> ()  [unwired: 1 out]
        n167 = property on="read gas flow" class="DigNum (strict)"("Value"=w351) -> ()  [unwired: 2 in, 2 out]
        n168 = call "data_headers_subVI_w_gases.vi"("Experiment Notes"=w299, "Sample names"=w311) -> ("data headers"=w310:string[])  [unwired: 9 in]
        n169 = Get Date/Time In Seconds() -> (seconds since 1Jan1904=w462:timestamp)
        n170 = Number To Engineering String ("elapsed time (min)")(4:w384) -> (0:w389:string)  [unwired: 3 in]
        n171 = Unbundle(w366) -> ("current  step # in"=w346:i32, "sequence end time in"=w365:timestamp, "Boolean"=w364:bool)
        n172 = Format Date/Time String(time format string (%c)="%Y-%m-%d %H:%M:%S%2u", seconds (now)=w462) -> (date/time string=w441:string)  [unwired: 1 in]
        n173 = Unbundle(w397) -> ("String data out"=w388:string, w387:string, w386:string, w385:string)
        n174 = Unbundle(w440) -> ("String"=w390:string, "String"=w443:string, "String"=w442:string)
        n175 = Unbundle(w381) -> ("String"=w380:string, "String"=w379:string)
        n176 = Unbundle(w355) -> ("pressure"=w435:string, "RH"=w434:string, "gas flow"=w433:string, "vapor flow"=w432:string)
        n177 = Unbundle ("arduino 1-6")(w340) -> ("mean"=w344:string, "mean"=w439:string, "mean"=w438:string, "mean"=w437:string, "mean"=w436:string, "mean"=w342:string)
        n178 = Increment(x=w346) -> (x+1=w345:i32)
        n179 = Build Array(w441, w389, w388, w387, w386, w385, w390, w443, w442, w380, w379, w435, w434, w433, w432, w343, w344, w439, w438, w437, w436, w342) -> (w449:string[])
        n180 = property on="Current\nstep" class="DigNum (strict)"("Value"=w345) -> ()  [unwired: 2 in, 2 out]
        "State date/time" <- w383
      }
      n181 = Unbundle(w90) -> (w89:bool, "VISA resource name out"=w88:refnum<visa-resource-name>, "error out"=w87:errorcluster)
      n182 = Unbundle(w86) -> ("Boolean"=w85:bool, "VISA out"=w84:refnum<visa-resource-name>, "error out"=w83:errorcluster)
      n183 = call-poly <vilib>:"Write To Spreadsheet File.vi"("1D data"=w55, "file path (dialog if empty)"=w71) -> ("new file path (Not A Path if cancelled)"=w75:path)  [unwired: 6 in]
      n184 = Unbundle(w64) -> (w69:bool, "VISA resource name out"=w68:refnum<visa-resource-name>, "error out"=w67:errorcluster)
      n185 = Unbundle(w37) -> ("Boolean"=w36:bool, "task out"=w19:refnum<k21>, "error out"=w18:errorcluster, "task out"=w17:refnum<k21>, "error out"=w16:errorcluster, "VISA resource name out"=w15:refnum<visa-resource-name>, "error out"=w14:errorcluster)
      n186 = call "arduino_close_subIV.vi"("arduino 1-6 addresses and errors out"=w57, "arduinos on?"=w56) -> ()  [unwired: 10 in]
      n187 = case shown="True" w49 {
        tunnel: w48 -> [_ w110]
        tunnel: w47 -> [w107 w109]
        tunnel: [w107 w108] -> w46
        frame False {
        }
        frame True {
          n188 = call "Close.vi"("VISA resource name"=w110, "error in (no error)"=w109) -> ("error out"=w108:errorcluster)  [unwired: 17 in]
        }
      }
      n189 = flat-sequence {
        tunnel: w24 -> [w106]
        tunnel: [w106] -> w23
        frame #0 {
          n190 = property on="saving data?" class="Bool (strict)"("Value"=FALSE ("saving data?")) -> ()  [unwired: 2 in, 2 out]
        }
      }
      n191 = Unbundle(w81) -> ("Boolean"=w80:bool, "VISA resource name out"=w79:refnum<visa-resource-name>, "error out"=w78:errorcluster)
      n192 = case shown="True" w36 {
        tunnel: [errorcluster {"status"=FALSE, "code"=0, "source"=""} ("error out") w135] -> w41
        tunnel: w19 -> [_ w134]
        tunnel: w18 -> [_ w133]
        tunnel: w17 -> [_ w132]
        tunnel: w16 -> [_ w129]
        tunnel: w15 -> [_ w130]
        tunnel: w14 -> [_ w131]
        tunnel: w10 -> [_ w126]
        tunnel: w9 -> [_ w125]
        frame False {
        }
        frame True {
          n193 = call <vilib>:"DAQmx Stop Task.vi"("task/channels in"=w134, "error in"=w133) -> ("task out"=w141:refnum<k21>, "error out"=w140:errorcluster)  [unwired: 12 in]
          n194 = call <vilib>:"DAQmx Stop Task.vi"("task/channels in"=w132, "error in"=w129) -> ("task out"=w142:refnum<k21>, "error out"=w143:errorcluster)  [unwired: 12 in]
          n195 = VISA Clear(VISA resource name=w130, error in (no error)=w131) -> (VISA resource name out=w139:refnum<visa-resource-name>, error out=w138:errorcluster)
          n196 = VISA Close(VISA resource name=w126, error in (no error)=w125) -> (error out=w127:errorcluster)
          n197 = VISA Close(VISA resource name=w139, error in (no error)=w138) -> (error out=w128:errorcluster)
          n198 = call <vilib>:"DAQmx Clear Task.vi"("task in"=w141, "error in"=w140) -> ("error out"=w137:errorcluster)  [unwired: 13 in]
          n199 = call <vilib>:"DAQmx Clear Task.vi"("task in"=w142, "error in"=w143) -> ("error out"=w136:errorcluster)  [unwired: 13 in]
          n200 = Merge Errors(w137, w136, w128, w127) -> (w135:errorcluster)
        }
      }
      n201 = case shown="True" w89 {
        tunnel: w88 -> [_ w259]
        tunnel: w87 -> [w256 w258]
        tunnel: [w256 w257] -> w91
        frame False {
        }
        frame True {
          n202 = call "Enable Output.vi"("error in (no error)"=w258, "Enable Output (T: Enable)"=FALSE, "VISA resource name"=w259) -> ("error out"=w260:errorcluster, "VISA resource name out"=w262:refnum<visa-resource-name>)  [unwired: 7 in]
          n203 = call "Close.vi"("error in (no error)"=w260, "VISA resource name"=w262) -> ("error out"=w257:errorcluster)  [unwired: 9 in]
        }
      }
      n204 = case shown="True" w69 {
        tunnel: w68 -> [_ w174]
        tunnel: w67 -> [w172 w173]
        tunnel: [w172 w175] -> w63
        frame False {
        }
        frame True {
          n205 = call "Enable Output.vi"("error in (no error)"=w173, "Enable Output (F:Off)"=FALSE ("Output (F:Off)"), "VISA resource name"=w174) -> ("error out"=w176:errorcluster, "VISA resource name out"=w177:refnum<visa-resource-name>)  [unwired: 7 out]
          n206 = call "Close.vi"("error in (no error)"=w176, "VISA resource name"=w177) -> ("error out"=w175:errorcluster)  [unwired: 9 out]
        }
      }
      n207 = case shown="True" w85 {
        tunnel: w83 -> [w242 w245]
        tunnel: [w242 w244] -> w92
        tunnel: w84 -> [_ w243]
        frame False {
        }
        frame True {
          n208 = call "srsQcm200Close.vi"("error in"=w245, "Visa in"=w243) -> ("error out"=w244:errorcluster)  [unwired: 3 in]
        }
      }
      n209 = call-poly <vilib>:"Write To Spreadsheet File.vi"("append to file? (new file:F)"=TRUE, "2D data"=w59, "file path (dialog if empty)"=w75) -> ()  [unwired: 5 in, 1 out]
      n210 = case shown="True" w80 {
        tunnel: w79 -> [_ w212]
        tunnel: w78 -> [w209 w211]
        tunnel: [w209 w210] -> w77
        frame False {
        }
        frame True {
          n211 = VISA Close(VISA resource name=w212, error in (no error)=w211) -> (error out=w210:errorcluster)
        }
      }
      n212 = Merge Errors(w63, w77, w91, w46, w92, w23) -> (w98:errorcluster)
      n213 = call <vilib>:"Simple Error Handler.vi"("error in (no error)"=w41) -> ()  [unwired: 4 in, 5 out]
      n214 = call <vilib>:"Simple Error Handler.vi"("error in (no error)"=w98) -> ()  [unwired: 4 in, 5 out]
    }
  }
